vi "set_increment.vi"(8 "error in (no error)":errorcluster, 9 "time increment":dbl[unit], 10 "z increment":dbl[unit], 11 "ImageCollection in":refnum<class "ImageCollection.lvclass">) -> (0 "error out":errorcluster, 3 "ImageCollection out":refnum<class "ImageCollection.lvclass">)   [LabVIEW 2010, in "ImageCollection.lvclass"]
uses:
  ImageCollection.lvclass
  type_enum.ctl
  ImageCollection.lvclass/ImageCollection.ctl
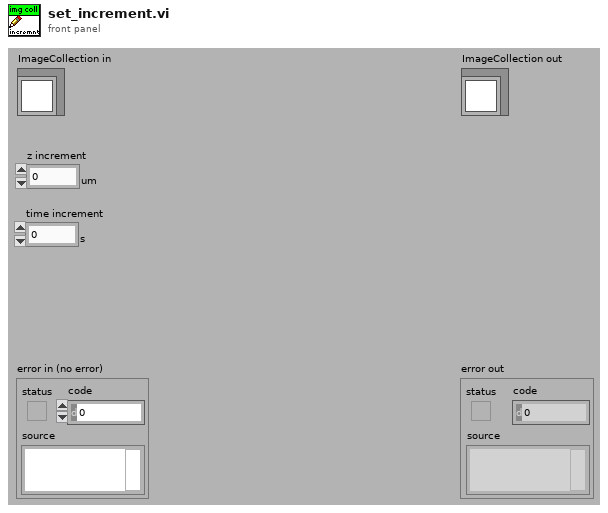
[diagram p1: front panel]
types:
  T1 = typedef "type_enum.ctl" = enum16{"undefined", "movie", "z-stack"}
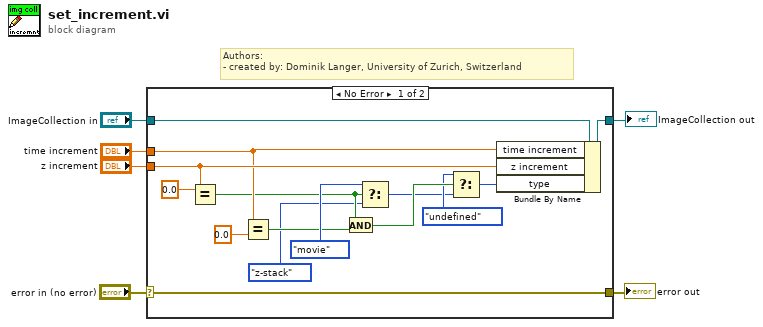
[diagram p0: block diagram]
diagram:
  # "Authors: \n- created by: Dominik Langer, University of Zurich, Switzerland"
  n1 = case shown="No Error" "error in (no error)" {
    selector: "error in (no error)" -> [w21 w23]
    tunnel: [w21 w23] -> w5
    tunnel: [w19 w22] -> w3
    tunnel: "ImageCollection in" -> [w20 w22]
    tunnel: "z increment" -> [w18 _]
    tunnel: "time increment" -> [w15 _]
    frame No Error {
      n2 = Equal?(x=dbl[unit] 0.0, y=w18) -> (x = y?=w12:bool)
      n3 = Equal?(x=w15, y=dbl[unit] 0.0) -> (x = y?=w13:bool)
      n4 = And(x=w12, y=w13) -> (x .and. y?=w11:bool)
      n5 = Select(t=type_enum."movie" ("type"), s=w12, f=type_enum."z-stack" ("type")) -> (s? t:f=w8:T1)
      n6 = Select(t=type_enum."undefined" ("type"), s=w11, f=w8) -> (s? t:f=w7:T1)
      n7 = Bundle By Name(cluster=w20, "time increment"=w15, "z increment"=w18, "type"=w7) -> (w19:refnum<class "ImageCollection.lvclass">)
    }
    frame Error {
    }
  }
  "error out" <- w5
  "ImageCollection out" <- w3
